vi "set64ChanHeader.vi"() -> (0 "64 Chan Header":string[](array[string]))   [LabVIEW 2013]
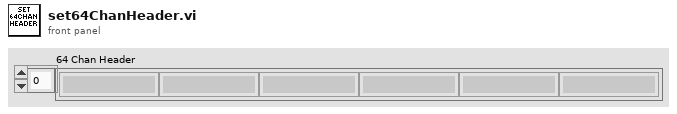
[diagram p1: front panel]
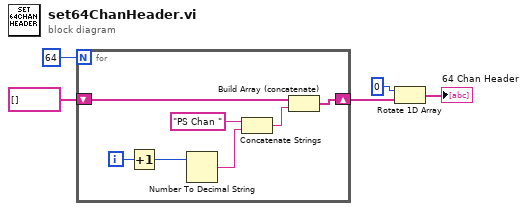
[diagram p0: block diagram]
diagram:
  n1 = for {
    N: 64 -> [_]
    shift-right: [w8] -> w3
    shift-left: string[] [] ("array") -> [w9]
    i -> [w7]
    n2 = Increment(x=w7) -> (x+1=w6:i32)
    n3 = Number To Decimal String(number=w6) -> (decimal integer string=w12:string)  [unwired: 1 in]
    n4 = Concatenate Strings("PS Chan " ("string"), w12) -> (w10:string)
    n5 = Build Array (concatenate)(w9, w10) -> (w8:string[])
  }
  n6 = Rotate 1D Array(1:w3, 2:0 ("n")) -> (0:→"64 Chan Header":string[])
